vi "Write Prefix.vi"(8 "error in (no error)":errorcluster, 10 "Prefix":string, 11 "Lakeshore 336 in":refnum<class "Lakeshore 336.lvclass">) -> (0 "error out":errorcluster, 3 "Lakeshore 336 out":refnum<class "Lakeshore 336.lvclass">)   [LabVIEW 2022 SP3, in "Lakeshore 336.lvclass"]
uses:
  Lakeshore 336.lvclass
  Lakeshore 336.lvclass/Lakeshore 336.ctl
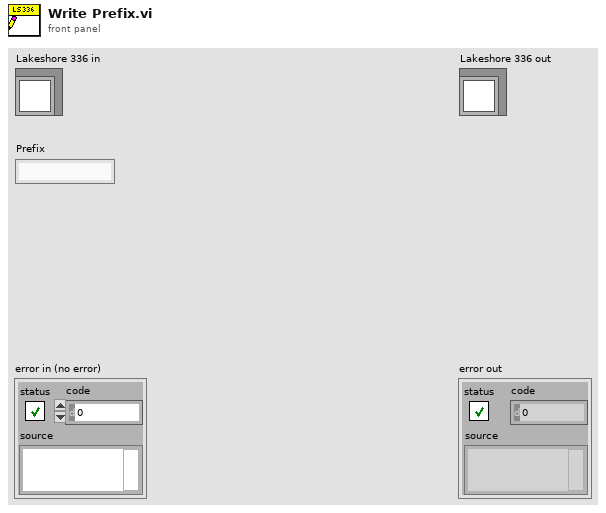
[diagram p1: front panel]
types:
  T1 = typedef "Lakeshore 336.lvclass/Lakeshore 336 Settings cluster.ctl" = cluster{"Lake Shore 336 Address":refnum<visa-resource-name>, "Output Ch":T2[], "Input Ch":T4[], "Prefix":string}
  T2 = typedef "Lakeshore 336.lvclass/Lakeshore 336 Channel Settings cluster.ctl" = cluster{"Input (0:None)":u16, "Power Up Enable (F: Off)":bool, "Mode (0:Off)":u16, "Max Current (0:User Specified)":u16, "Heater Out Display (1:Current)":u16, "Max User Current (2.000)":dbl, "Heater Resistance (1:25 Ohms)":u16, "PID":T3, "Name":string}
  T3 = typedef "Lakeshore 336.lvclass/Lakeshore 336 PID cluster.ctl" = cluster{"P":dbl, "I":dbl, "D":dbl}
  T4 = typedef "Lakeshore 336.lvclass/Lakeshore 336 Input Ch config cluster.ctl" = cluster{"Name":string}
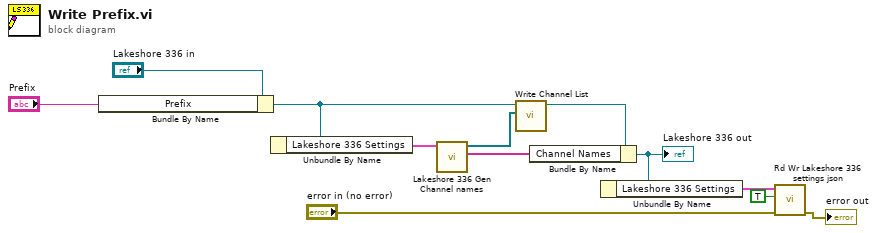
[diagram p0: block diagram]
diagram:
  n1 = Bundle By Name(cluster="Lakeshore 336 in", "Prefix"="Prefix") -> (w11:refnum<class "Lakeshore 336.lvclass">)
  n2 = Unbundle By Name(w11) -> ("Lakeshore 336 Settings"=w12:T1)
  n3 = call "Lakeshore 336 Gen Channel names.vi"("Lakeshore 336 Settings"=w12) -> ("Channel Names"=w8:string[], "Channel List"=w10:refnum<class "HK Item.lvclass">[])  [unwired: 9 in]
  n4 = call-dynamic "Write Channel List.vi"("Channel List"=w10, "Temp Control in"=w11) -> ("Temp Control out"=w9:refnum<class "Lakeshore 336.lvclass">)  [unwired: 8 in, 1 out]
  n5 = Bundle By Name(cluster=w9, "Channel Names"=w8) -> (w7:refnum<class "Lakeshore 336.lvclass">)
  "Lakeshore 336 out" <- w7
  n6 = Unbundle By Name(w7) -> ("Lakeshore 336 Settings"=w6:T1)
  n7 = call "Rd Wr Lakeshore 336 settings json.vi"("error in (no error)"="error in (no error)", "Write? (F:Read)"=TRUE, "Lakeshore 336 Settings"=w6) -> ("error out"=→"error out":errorcluster)  [unwired: 7 in, 1 out]
